vi "KE_Acquire.vi"(6 "Boolean":bool=TRUE, 7 "Type":u16(ring) items=["First", "Second", "Init"], 8 "error in (no error)":errorcluster, 11 "Instruments in":refnum<class "Instruments.lvclass">) -> (0 "error out":errorcluster, 3 "Instruments out":refnum<class "Instruments.lvclass">, 5 "Voltage":dbl)   [LabVIEW 2012, in "Instruments.lvclass"]
uses:
  Instruments.lvclass
  Instruments.lvclass/Instruments.ctl
  Instruments/Drivers/ke236/KE236.LLB/Keith 236 Operate/Standby.vi
panel:
  in  "integration time (medium:1)":u16(ring)=1 items=["fast perod", "medium period", "line cycle period @ 50Hz", "line cycle period @ 60Hz"]
  out "device dependent errors":string
  out "?":T1(array[cluster])
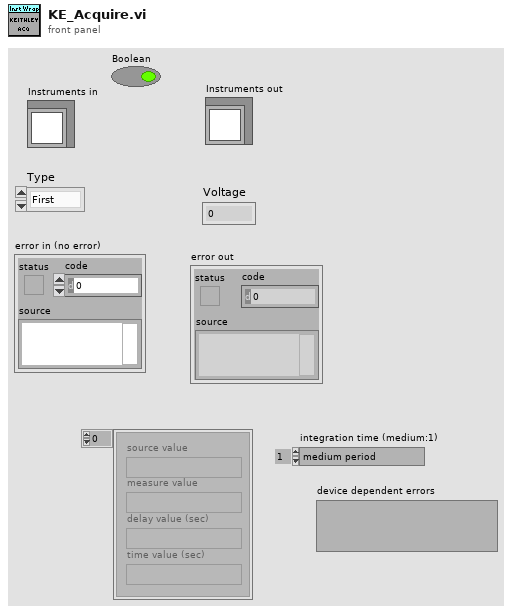
[diagram p1: front panel]
types:
  T1 = cluster{"source value":string, "measure value":string, "delay value (sec)":string, "time value (sec)":string}[]
  T2 = cluster{"Start Current,mA":dbl, "Stop Current,mA":dbl, "Voltage Compliance,V":dbl, "GPIB":string}
  T3 = cluster{"error":bool, "code":i32, "source":string}
  T4 = cluster{"source value":string, "measure value":string, "delay value (sec)":string, "time value (sec)":string}
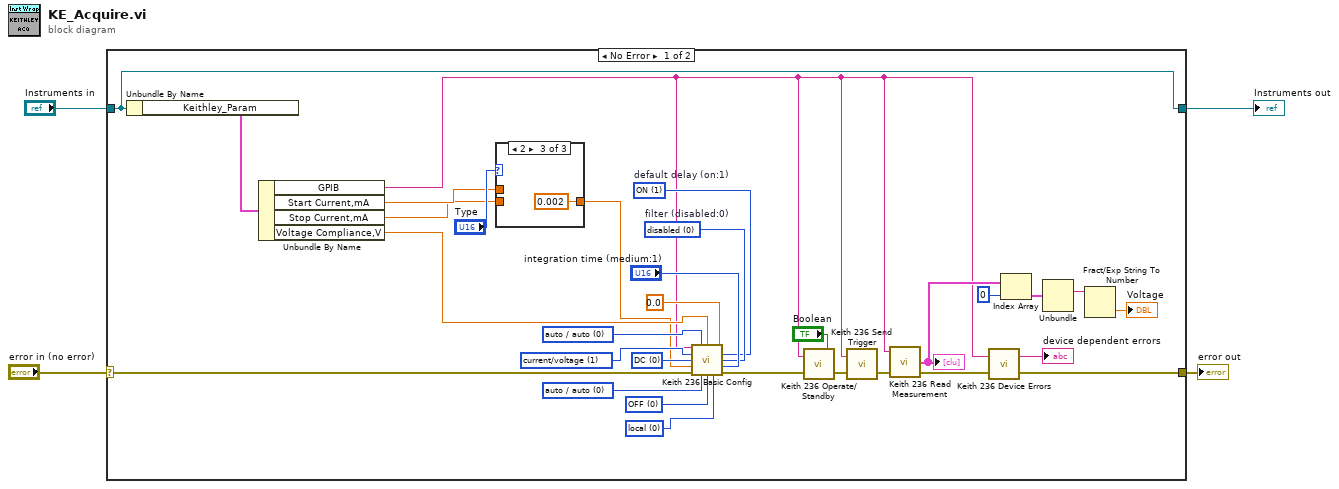
[diagram p0: block diagram]
diagram:
  n1 = case shown="No Error" "error in (no error)" {
    selector: "error in (no error)" -> [w6 w40]
    tunnel: [w8 w40] -> w3
    tunnel: [w7 w39] -> w1
    tunnel: "Instruments in" -> [w7 w39]
    frame No Error {
      w21 = u16 1 items=["OFF", "ON"]  # default delay (on:1)
      w22 = u16 0 items=["disabled", "2 readings", "4 readings", "8 readings", "16 readings", "32 readings"]  # filter (disabled:0)
      w25 = u16 0 items=["local", "remote"] ("sense (local:0)")
      w26 = u16 0 items=["OFF", "ON"] ("suppression (off:0)")
      w27 = u16 0 items=["auto / auto", "1 nA / 1.1 V", "10 nA / 11 V", "100 nA / 110 V", "0.001 mA / 110 V", "0.01 mA / 110 V", "0.1 mA / 110 V", "1 mA / 110 V", "10 mA / 110 V", "100 mA / 110 V"] ("compliance/\nmeasurement range (auto:0)")
      w28 = u16 0 items=["DC", "sweep"] ("function (DC:0)")
      w29 = u16 1 items=["voltage/current", "current/voltage"] ("source/measure (V/I:0)")
      w30 = u16 0 items=["auto / auto", "1 nA / 1.1 V", "10 nA / 11 V", "100 nA / 110 V", "0.001 mA / 110 V", "0.01 mA / 110 V", "0.1 mA / 110 V", "1 mA / 110 V", "10 mA / 110 V", "100 mA / 110 V"] ("source range\nI source / V source (auto:0)")
      n2 = Unbundle By Name(w7) -> ("Keithley_Param"=w5:T2)
      n3 = Unbundle By Name(w5) -> ("GPIB"=w13:string, "Start Current,mA"=w11:dbl, "Stop Current,mA"=w10:dbl, "Voltage Compliance,V"=w20:dbl)
      n4 = case shown="2" "Type" {
        tunnel: w11 -> [w36 _ _]
        tunnel: w10 -> [_ w37 _]
        tunnel: [w36 w37 0.002 ("Stop Current,mA")] -> w9
        frame 0, Default {
        }
        frame 1 {
        }
        frame 2 {
        }
      }
      n5 = call "Keith 236 Basic Config.vi"("GPIB address"=w13, "source range\nI source / V source (auto:0)"=w30, "voltage \ncompliance level"=w20, "DC delay (sec)"=0.0, "source/measure (V/I:0)"=w29, "default delay (on:1)"=w21, "function (DC:0)"=w28, "filter (disabled:0)"=w22, "source level"=w9, "integration time (medium:1)"="integration time (medium:1)", "error in"=w6, "compliance/\nmeasurement range (auto:0)"=w27, "suppression (off:0)"=w26, "sense (local:0)"=w25) -> ("error out"=w19:T3)  [unwired: 1 in]
      n6 = call "Keith 236 Operate/Standby.vi"("source"="Boolean", "error in"=w19, "GPIB address"=w13) -> ("error out"=w32:T3)
      n7 = call "Keith 236 Send Trigger.vi"("GPIB address"=w13, "error in"=w32) -> ("error out"=w34:T3)
      n8 = call "Keith 236 Read Measurement.vi"("error in"=w34, "GPIB address"=w13) -> ("error out"=w35:T3, "display"=w18:T1)  [unwired: 2 out]
      "?" <- w18
      n9 = call "Keith 236 Device Errors.vi"("error in"=w35, "GPIB address"=w13) -> ("error out"=w8:T3, "device dependent errors"=→"device dependent errors":string)
      n10 = Index Array(array=w18, index=0) -> (element=w16:T4)
      n11 = Unbundle(w16) -> ("measure value"=w15:string)  [unwired: 3 out]
      n12 = Fract/Exp String To Number(string=w15) -> (number=→"Voltage":dbl)  [unwired: 3 in, 1 out]
    }
    frame Error {
    }
  }
  "error out" <- w3
  "Instruments out" <- w1
